vi "check victory (subvi).vi"(9 "Игрок":i32, 10 "Игровое поле":i32[][](array[ring]) items=["", "X", "0"]) -> (4 "Победа":bool)   [LabVIEW 2017]
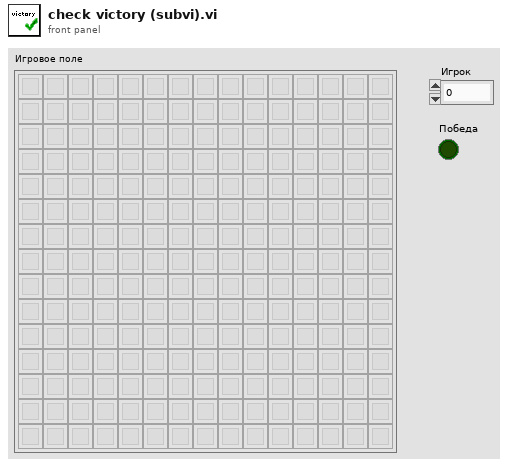
[diagram p1: front panel]
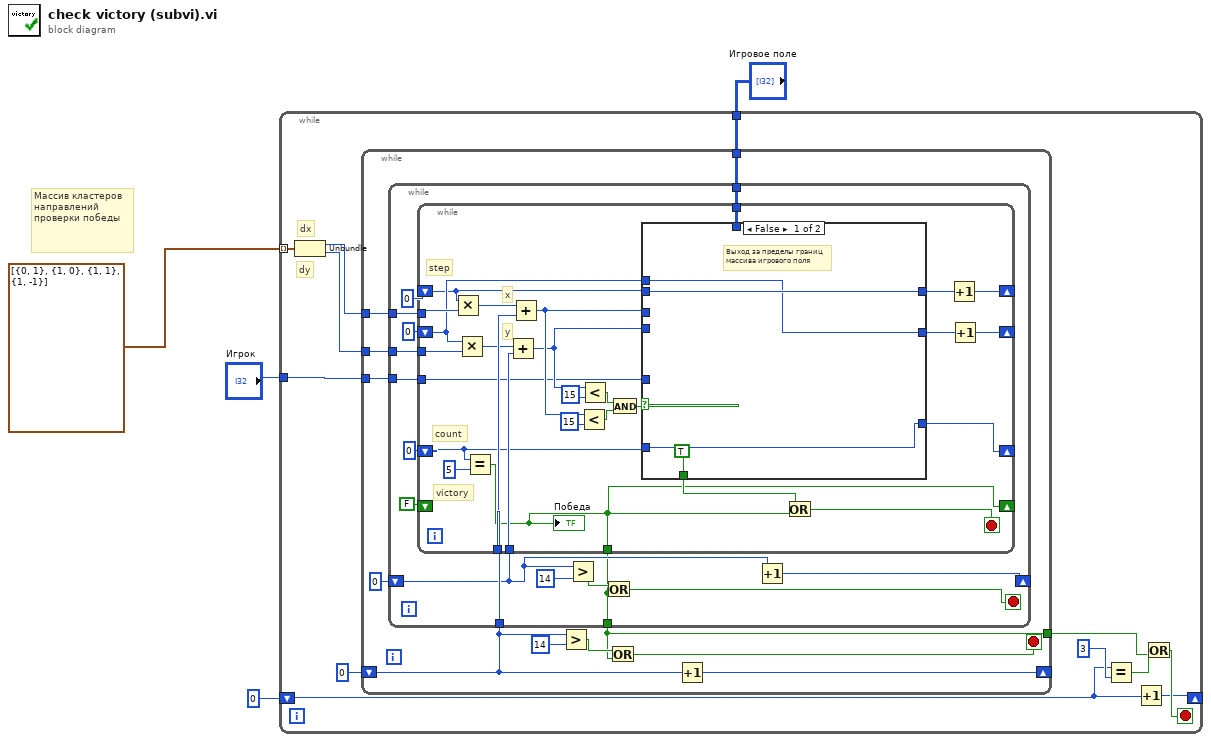
[diagram p0: block diagram]
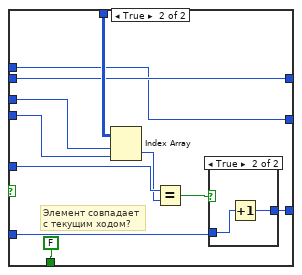
[diagram p2: hidden frame]
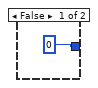
[diagram p3: hidden frame]
diagram:
  # "Массив кластеров направлений проверки победы"
  n1 = while {
    tunnel: cluster{i32, i32}[] [{0, 1}, {1, 0}, {1, 1}, {1, -1}] -> [w16] mode=indexing
    tunnel: "Игровое поле" -> [w14]
    tunnel: "Игрок" -> [w12]
    shift-right: [w8] -> _
    shift-left: 0 -> [w5]
    stop <- w9 stop-if-true
    # "dy"
    # "dx"
    n2 = Unbundle(w16) -> (w15:i32, w13:i32)
    n3 = while {
      tunnel: w15 -> [w19]
      tunnel: w14 -> [w27]
      tunnel: w13 -> [w26]
      tunnel: w12 -> [w25]
      shift-right: [w21] -> _
      shift-left: 0 -> [w17]
      tunnel: [w18] -> w6
      stop <- w22 stop-if-true
      n4 = while {
        tunnel: w17 -> [w42]
        tunnel: w27 -> [w39]
        tunnel: w26 -> [w41]
        tunnel: w25 -> [w40]
        shift-right: [w33] -> _
        shift-left: 0 -> [w34]
        tunnel: w19 -> [w30]
        tunnel: [w28] -> w18
        stop <- w35 stop-if-true
        n5 = while {
          shift-right: [w69] -> _
          shift-left: 0 -> [w46]
          tunnel: w42 -> [w67]
          shift-right: [w54] -> _
          shift-left: 0 -> [w47]
          tunnel: w41 -> [w66]
          tunnel: w34 -> [w64]
          tunnel: w40 -> [w49]
          tunnel: w39 -> [w58]
          shift-right: [w52] -> _
          shift-left: 0 -> [w51]
          tunnel: w30 -> [w48]
          shift-right: [w43] -> _
          shift-left: FALSE -> [_]
          tunnel: [w43] -> w28
          stop <- w44 stop-if-true
          # "victory"
          # "count"
          # "y"
          # "x"
          # "step"
          n6 = Multiply(x=w46, y=w48) -> (x*y=w68:i32)
          n7 = Multiply(x=w47, y=w66) -> (x*y=w65:i32)
          n8 = Equal?(x=w51, y=5) -> (x = y?=w43:bool)
          "Победа" <- w43
          n9 = Add(x=w65, y=w64) -> (x+y=w56:i32)
          n10 = Add(x=w68, y=w67) -> (x+y=w57:i32)
          n11 = Less?(x=w57, y=15) -> (x < y?=w59:bool)
          n12 = Less?(x=w56, y=15) -> (x < y?=w60:bool)
          n13 = And(x=w60, y=w59) -> (x .and. y?=w61:bool)
          n14 = case shown="False" w61 {
            tunnel: w49 -> [_ w84]
            tunnel: w58 -> [_ w83]
            tunnel: w57 -> [_ w82]
            tunnel: w56 -> [_ w77]
            tunnel: [w71 w75] -> w55
            tunnel: w46 -> [w71 w75]
            tunnel: w47 -> [w70 w74]
            tunnel: [w70 w74] -> w53
            tunnel: [w72 w79] -> w52
            tunnel: w51 -> [w72 w78]
            tunnel: [TRUE FALSE] -> w45
            frame False {
              # "Выход за пределы границ\nмассива игрового поля"
            }
            frame True {
              # "Элемент совпадает с текущим ходом?"
              n15 = Index Array(array=w83, index (row)=w82, index (col)=w77) -> (element=w81:i32)
              n16 = Equal?(x=w84, y=w81) -> (x = y?=w80:bool)
              n17 = case shown="True" w80 {
                tunnel: [0 w87] -> w79
                tunnel: w78 -> [_ w86]
                frame False {
                }
                frame True {
                  n18 = Increment(x=w86) -> (x+1=w87:i32)
                }
              }
            }
          }
          n19 = Or(x=w45, y=w43) -> (x .or. y?=w44:bool)
          n20 = Increment(x=w55) -> (x+1=w69:i32)
          n21 = Increment(x=w53) -> (x+1=w54:i32)
        }
        n22 = Greater?(x=w34, y=14) -> (0:w36:bool)
        n23 = Or(x=w36, y=w28) -> (x .or. y?=w35:bool)
        n24 = Increment(x=w34) -> (x+1=w33:i32)
      }
      n25 = Greater?(x=w17, y=14) -> (0:w23:bool)
      n26 = Or(x=w23, y=w18) -> (x .or. y?=w22:bool)
      n27 = Increment(x=w17) -> (x+1=w21:i32)
    }
    n28 = Equal?(x=w5, y=3) -> (x = y?=w10:bool)
    n29 = Increment(x=w5) -> (x+1=w8:i32)
    n30 = Or(x=w10, y=w6) -> (x .or. y?=w9:bool)
  }
